vi "System Options.vi"(4 "Display Intensity (2)":i32=2, 5 "Beeper Volume (25)":dbl=25.0 format="%.2f", 6 "Key Lock (F:Unlocked)":bool, 7 "Key Beep (F:Off)":bool, 8 "error in (no error)":errorcluster, 10 "Display Update (T:Auto)":bool=TRUE, 11 "VISA resource name":refnum<visa-resource-name>) -> (0 "error out":errorcluster, 3 "VISA resource name out":refnum<visa-resource-name>)   [LabVIEW 2020, in "Berkeley Nucleonics 500 Series.lvlib"]
doc: "This VI is used to configure the display and keyboard atributes."
uses:
  Berkeley Nucleonics 500 Series.lvlib
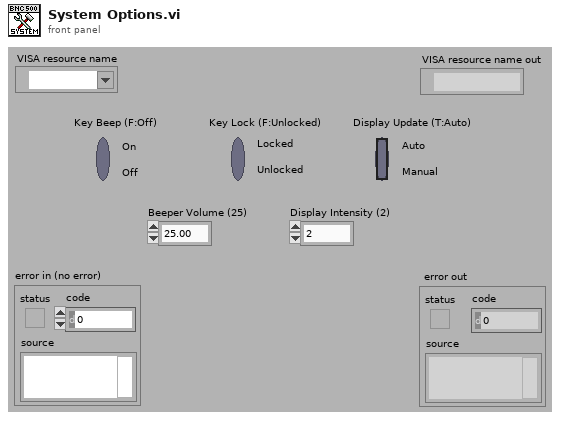
[diagram p1: front panel]
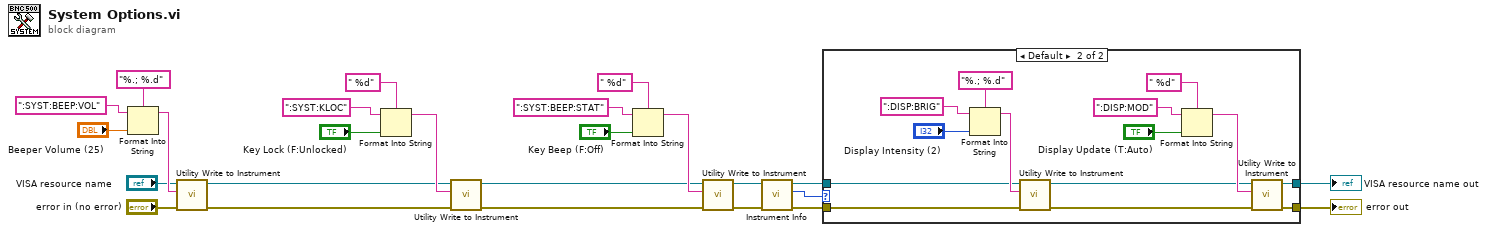
[diagram p0: block diagram]
diagram:
  n1 = Format Into String(format string="%.; %.d", initial string=":SYST:BEEP:VOL", "Beeper Volume (25)") -> (resulting string=w23:string)  [unwired: 1 in, 1 out]
  n2 = call "Utility Write to Instrument.vi"("error in (no error)"="error in (no error)", "Write Buffer"=w23, "VISA resource name"="VISA resource name") -> ("error out"=w3:errorcluster, "VISA resource name out"=w4:refnum<visa-resource-name>)  [unwired: 6 in, 1 out]
  n3 = Format Into String(format string=" %d", initial string=":SYST:KLOC", "Key Lock (F:Unlocked)") -> (resulting string=w18:string)  [unwired: 1 in, 1 out]
  n4 = call "Utility Write to Instrument.vi"("error in (no error)"=w3, "Write Buffer"=w18, "VISA resource name"=w4) -> ("error out"=w11:errorcluster, "VISA resource name out"=w12:refnum<visa-resource-name>)  [unwired: 6 in, 1 out]
  n5 = Format Into String(format string=" %d", initial string=":SYST:BEEP:STAT", "Key Beep (F:Off)") -> (resulting string=w15:string)  [unwired: 1 in, 1 out]
  n6 = call "Utility Write to Instrument.vi"("error in (no error)"=w11, "Write Buffer"=w15, "VISA resource name"=w12) -> ("error out"=w8:errorcluster, "VISA resource name out"=w7:refnum<visa-resource-name>)  [unwired: 6 in, 1 out]
  n7 = call "Instrument Info.vi"("error in (no error)"=w8, "VISA resource name"=w7) -> ("error out"=w5:errorcluster, "Instr Model"=w1:u32, "VISA resource name out"=w6:refnum<visa-resource-name>)  [unwired: 6 in, 1 out]
  n8 = case shown="Default" w1 {
    tunnel: [w26 w38] -> w9
    tunnel: w6 -> [w27 w33]
    tunnel: w5 -> [w26 w32]
    tunnel: [w27 w29] -> w2
    frame 505, 9610 {
    }
    frame Default {
      n9 = Format Into String(format string="%.; %.d", initial string=":DISP:BRIG", "Display Intensity (2)") -> (resulting string=w35:string)  [unwired: 1 in, 1 out]
      n10 = call "Utility Write to Instrument.vi"("error in (no error)"=w32, "Write Buffer"=w35, "VISA resource name"=w33) -> ("error out"=w31:errorcluster, "VISA resource name out"=w30:refnum<visa-resource-name>)  [unwired: 6 in, 1 out]
      n11 = Format Into String(format string=" %d", initial string=":DISP:MOD", "Display Update (T:Auto)") -> (resulting string=w39:string)  [unwired: 1 in, 1 out]
      n12 = call "Utility Write to Instrument.vi"("error in (no error)"=w31, "Write Buffer"=w39, "VISA resource name"=w30) -> ("error out"=w38:errorcluster, "VISA resource name out"=w29:refnum<visa-resource-name>)  [unwired: 6 in, 1 out]
    }
  }
  "error out" <- w9
  "VISA resource name out" <- w2
